vi "Set Metrics Min-Max.vi"(8 "error in (no error)":errorcluster, 10 "d_values":cluster{"min":dbl[], "max":dbl[]}, 11 "MF3 in":refnum<class "MF3.lvclass">) -> (0 "error out":errorcluster, 3 "MF3 out":refnum<class "MF3.lvclass">)   [LabVIEW 2011, in "MF3.lvclass"]
uses:
  MF3.lvclass
  MF3.lvclass/MF3.ctl
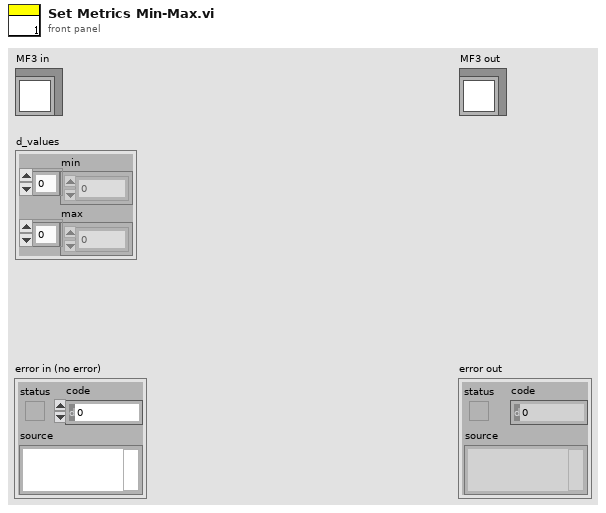
[diagram p1: front panel]
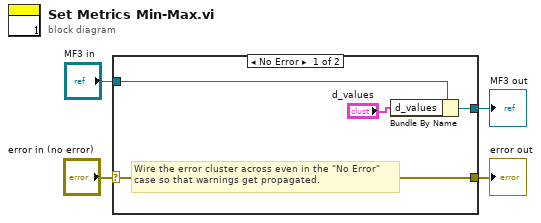
[diagram p0: block diagram]
diagram:
  n1 = case shown="No Error" "error in (no error)" {
    selector: "error in (no error)" -> [w8 w10]
    tunnel: [w8 w10] -> w3
    tunnel: [w6 w9] -> w1
    tunnel: "MF3 in" -> [w7 w9]
    frame No Error {
      # "Wire the error cluster across even in the \"No Error\"\ncase so that warnings get propagated."
      n2 = Bundle By Name(cluster=w7, "d_values"="d_values") -> (w6:refnum<class "MF3.lvclass">)
    }
    frame Error {
    }
  }
  "error out" <- w3
  "MF3 out" <- w1
